vi "Example.vi"() -> ()   [LabVIEW 2020, in "lvzstd.lvlib"]
uses:
  lvzstd.lvlib
panel:
  out "uncompressed":string="Test data"
  in  "data in":string="Test data"
  out "compressed data":string
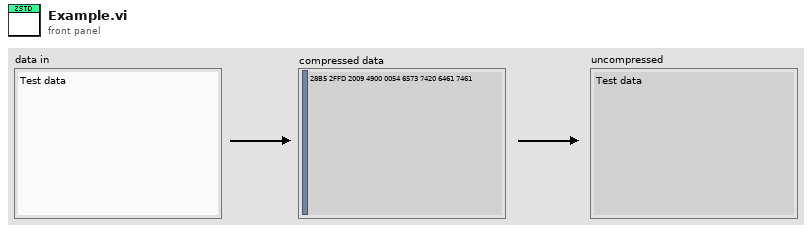
[diagram p1: front panel]
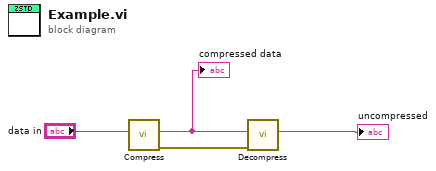
[diagram p0: block diagram]
diagram:
  n1 = call "Compress.vi"("data in"="data in") -> ("error out"=w4:errorcluster, "compressed data"=w2:string)  [unwired: 9 in]
  "compressed data" <- w2
  n2 = call "Decompress.vi"("error in (no error)"=w4, "compressed data"=w2) -> ("uncompressed data"=→"uncompressed":string)  [unwired: 8 in, 1 out]
